vi "test Remove Invalid Alias.vi"(8 "error in (no error)":errorcluster, 11 "TestCase in":refnum<class "Routing and Faulting Aliases Unit Tests.lvclass">) -> (0 "error out":errorcluster, 3 "TestCase out":refnum<class "Routing and Faulting Aliases Unit Tests.lvclass">)   [LabVIEW 2020, in "Routing and Faulting Aliases Unit Tests.lvclass"]
uses:
  Routing and Faulting Aliases Unit Tests.lvclass
  System Explorer/Alias.ctl
  System Explorer/Endpoint.ctl
  Shared/Alias Mapping.ctl
  Shared/Alias Endpoint.ctl
  Routing and Faulting Aliases Unit Tests.lvclass/Routing and Faulting Aliases Unit Tests.ctl
  <vilib>/addons/_JKI Toolkits/VI Tester/TestCase.llb/TestCase.lvclass
  System Explorer/Routing and Faulting System Explorer.lvlib
  Scripting/Routing and Faulting Scripting.lvlib
  Shared/Routing and Faulting Shared.lvlib
  C:/Program Files (x86)/National Instruments/LabVIEW 2020/vi.lib/addons/_JKI Toolkits/VI Tester/TestCase.llb/TestCase.lvclass
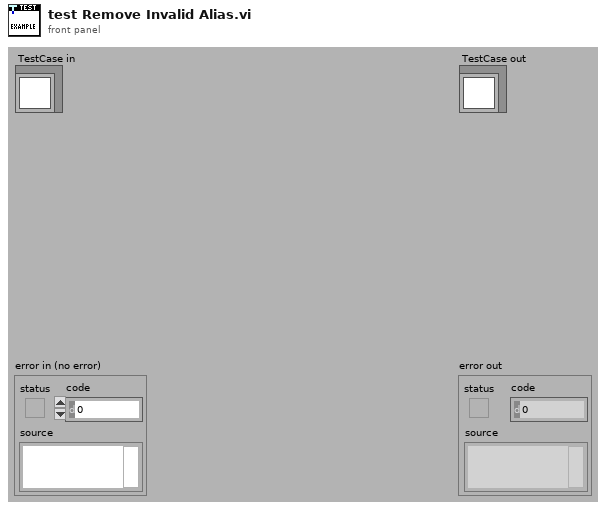
[diagram p1: front panel]
types:
  T1 = typedef "Routing and Faulting System Explorer.lvlib/Endpoint.ctl" = string
  T2 = typedef "Routing and Faulting Shared.lvlib/Alias Endpoint.ctl" = cluster{"Module Path":string, "Endpoint":string}
  T3 = typedef "Routing and Faulting Shared.lvlib/Alias Mapping.ctl" = cluster{"Alias":string, "Endpoint":T2}
  T4 = typedef "Routing and Faulting System Explorer.lvlib/Alias.ctl" = cluster{"Endpoint":T1, "Alias":string, "Remove":bool}
  T5 = typedef "Custom Device API.lvlib/Custom Device Item Ref.ctl" = u64
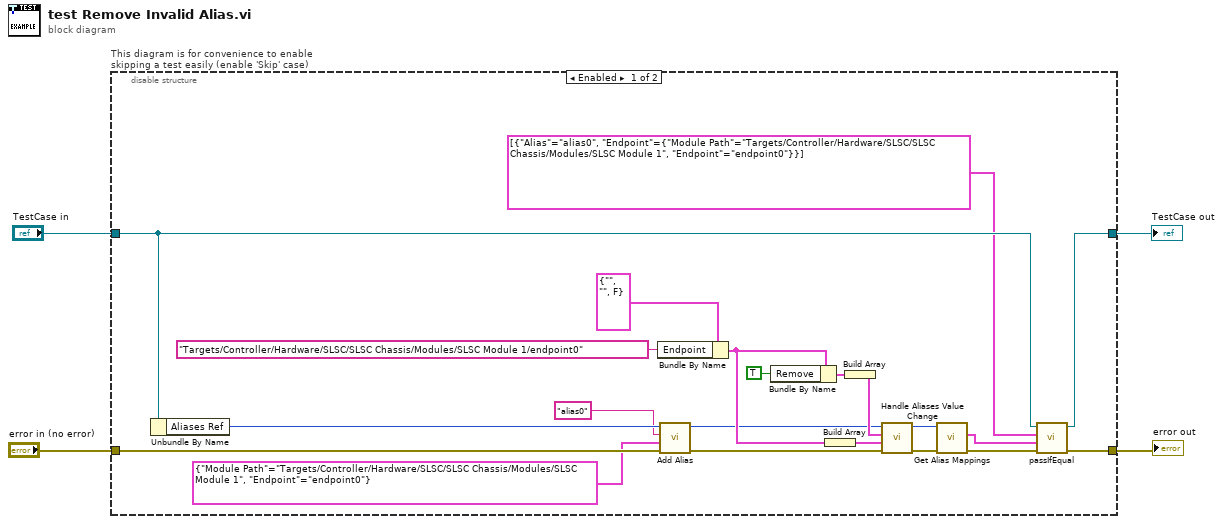
[diagram p0: block diagram]
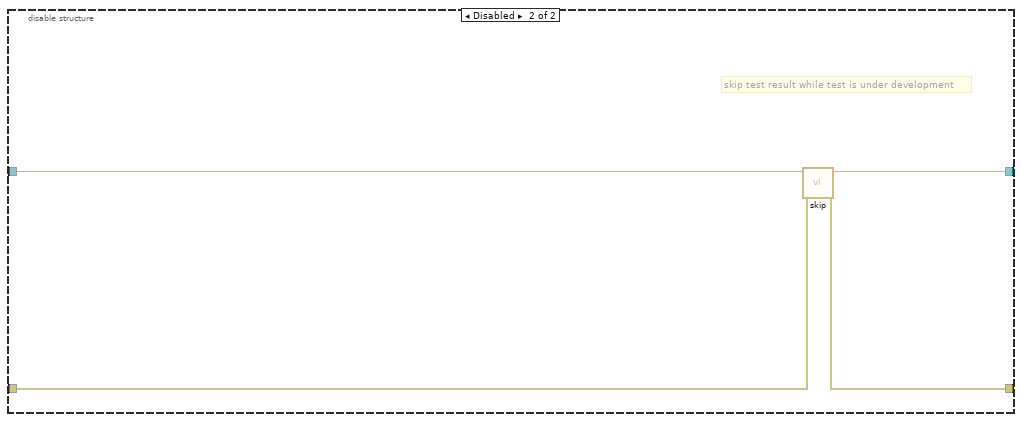
[diagram p2: hidden frame]
diagram:
  n1 = disable-structure "This diagram is for convenience to enable skipping a test easily (enable 'Skip' case)" shown="Enabled" {
    disable-tunnel: "TestCase in" -> [w22 w29]
    disable-tunnel: [w8 w27] -> w1
    disable-tunnel: [w11 w28] -> w3
    disable-tunnel: "error in (no error)" -> [w21 w26]
    frame Enabled {
      n2 = Unbundle By Name(w22) -> ("Aliases Ref"=w20:T5)
      n3 = Bundle By Name(cluster=T4 {"Endpoint"="", "Alias"="", "Remove"=FALSE} ("Alias"), "Endpoint"=T1 "Targets/Controller/Hardware/SLSC/SLSC Chassis/Modules/SLSC Module 1/endpoint0") -> (w15:T4)
      n4 = call "Add Alias.vi"("error in"=w21, "endpoint"=T2 {"Module Path"="Targets/Controller/Hardware/SLSC/SLSC Chassis/Modules/SLSC Module 1", "Endpoint"="endpoint0"} ("Endpoint"), "alias"="alias0" ("Alias"), "endpoint aliases in"=w20) -> ("error out"=w19:errorcluster, "endpoint aliases out"=w13:T5)  [unwired: 6 in]
      n5 = Bundle By Name(cluster=w15, "Remove"=TRUE) -> (w17:T4)
      n6 = Build Array(w15) -> (w14:T4[])
      n7 = Build Array(w17) -> (w16:T4[])
      n8 = call "Handle Aliases Value Change.vi"("error in (no error)"=w19, "OldVal"=w14, "NewVal"=w16, "Aliases Ref in"=w13) -> ("error out"=w25:errorcluster, "Aliases Ref out"=w24:T5)  [unwired: 4 in, 2 out]
      n9 = call "Get Alias Mappings.vi"("error in"=w25, "endpoint aliases in"=w24) -> ("error out"=w23:errorcluster, "alias mappings"=w12:T3[])  [unwired: 7 in, 1 out]
      n10 = call-dynamic "passIfEqual.vi"("error in (no error)"=w23, "y"=w12, "x"=T3[] [{"Alias"="alias0", "Endpoint"={"Module Path"="Targets/Controller/Hardware/SLSC/SLSC Chassis/Modules/SLSC Module 1", "Endpoint"="endpoint0"}}] ("Alias Mappings"), "TestCase in"=w22) -> ("error out"=w11:errorcluster, "TestCase out"=w8:refnum<class "Routing and Faulting Aliases Unit Tests.lvclass">)  [unwired: 6 in]
    }
    frame Disabled {
      # "skip test result while test is under development"
      n11 = call <vilib>:"skip.vi"("error in (no error)"=w26, "TestCase in"=w29) -> ("error out"=w28:errorcluster, "TestCase out"=w27:refnum<class "Routing and Faulting Aliases Unit Tests.lvclass">)  [unwired: 8 in]
    }
  }
  "error out" <- w3
  "TestCase out" <- w1
